vi "insertKeyInLogFile.vi"(10 "RFID_log_file_path":path, 11 "trimmed string":string) -> ()   [LabVIEW 2024]
uses:
  <vilib>/Utility/file.llb/Read Delimited Spreadsheet (string).vi
  <vilib>/Utility/file.llb/Write Delimited Spreadsheet (string).vi
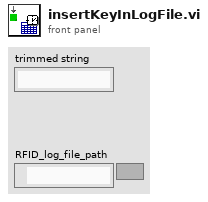
[diagram p1: front panel]
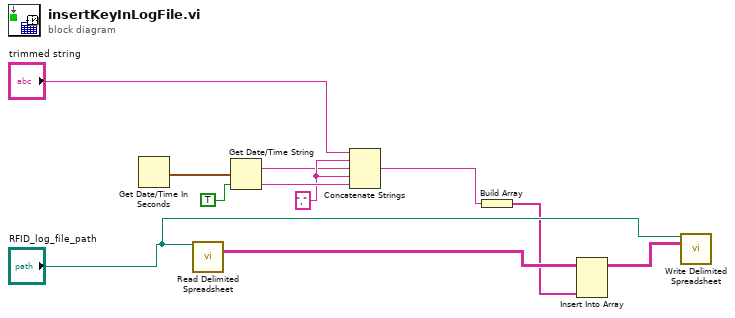
[diagram p0: block diagram]
diagram:
  w7 = "," ("string")
  n1 = Get Date/Time In Seconds() -> (seconds since 1Jan1904=w1:timestamp)
  n2 = call-poly <vilib>:"Read Delimited Spreadsheet.vi"("file path (dialog if empty)"="RFID_log_file_path") -> ("all rows"=w4:string[][])  [unwired: 9 in, 5 out]
  n3 = Get Date/Time String(seconds (now)=w1, want seconds? (F)=TRUE) -> (date string=w6:string, time string=w8:string)  [unwired: 1 in]
  n4 = Concatenate Strings("trimmed string", w7, w6, w7, w8) -> (w9:string)
  n5 = Build Array(w9) -> (w3:string[])
  n6 = Insert Into Array(array=w4, new element=w3) -> (w11:string[][])  [unwired: 2 in]
  n7 = call-poly <vilib>:"Write Delimited Spreadsheet.vi"("file path (dialog if empty)"="RFID_log_file_path", "2D data"=w11) -> ()  [unwired: 12 in, 2 out]
